vi "EN50160 Aggregation.vi"   [LabVIEW 2014, in "NI_EP_Power Quality.lvlib"]
doc: "Calculates aggregated values of power quality parameters for specific intervals. You use the aggregated values for further evaluations according to EN 50160:2007. The aggregation methods are compliant with Class S in IEC 61000-4-30:2008. The aggregation is based on a 10-cycle time interval for a 50 Hz power system or 12-cycle time interval for a 60 Hz power system. There is no overlap between aggregation intervals. This VI automatically restarts accumulation at the beginning of the next 10/12-cycle time interval after the previous interval expires. You must manually select the polymorphic instance you want to use.\n\nThis VI supports measuring single-bus single-line or multiple-bus single-line systems."
uses:
  <vilib>/addons/Electrical Power/PQ/NI_EP_Power Quality.lvlib
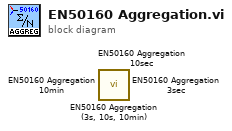
[diagram p0: block diagram]
diagram:
  n1 = call <vilib>:"EN50160 Aggregation (3s, 10s, 10min).vi"() -> ()  [unwired: 15 in, 5 out]
  n2 = call <vilib>:"EN50160 Aggregation 10sec.vi"() -> ()  [unwired: 17 in, 3 out]
  n3 = call <vilib>:"EN50160 Aggregation 10min.vi"() -> ()  [unwired: 17 in, 3 out]
  n4 = call <vilib>:"EN50160 Aggregation 3sec.vi"() -> ()  [unwired: 17 in, 3 out]
